vi "7.vi"(11 "文字列入力":string) -> (3 "文字列出力":string)   [LabVIEW 2019]
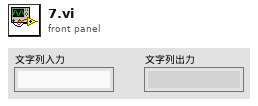
[diagram p1: front panel]
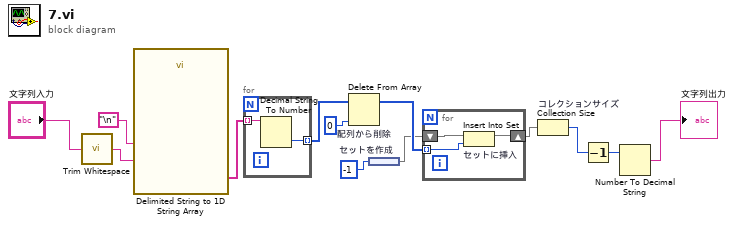
[diagram p0: block diagram]
diagram:
  n1 = call <vilib>:"Trim Whitespace.vi"("string"="文字列入力") -> ("trimmed string"=w6:string)  [unwired: 1 in]
  n2 = call <vilib>:"Delimited String to 1D String Array.vi"("delimiter"="\n", "delimited string"=w6) -> ("string array"=w9:string[])  [unwired: 9 in]
  n3 = for {
    tunnel: w9 -> [w15] mode=indexing
    tunnel: [w14] -> w10 mode=indexing
    n4 = Decimal String To Number(string=w15) -> (number=w14:i32)  [unwired: 2 in, 1 out]
  }
  n5 = Delete From Array "配列から削除"(array=w10, index=0) -> (array with subset deleted=w5:i32[])  [unwired: 1 in, 1 out]
  n6 = node "セットを作成"(-1) -> (w4:set{i32})
  n7 = for {
    tunnel: w5 -> [w17] mode=indexing
    shift-right: [w16] -> w2
    shift-left: w4 -> [w18]
    n8 = Insert Into Set "セットに挿入"(10:w17, 11:w18) -> (3:w16:set{i32})  [unwired: 1 out]
  }
  n9 = Collection Size "コレクションサイズ"(1:w2) -> (0:w11:i32)
  n10 = Decrement(x=w11) -> (x-1=w1:i32)
  n11 = Number To Decimal String(number=w1) -> (decimal integer string=→"文字列出力":string)  [unwired: 1 in]
